vi "init.vi"(8 "error in (no error)":errorcluster, 9 "Image Type":T1=1 items=["Grayscale (U8)", "Grayscale (I16)", "Grayscale (SGL)", "Complex (CSG)", "RGB (U32)", "HSL (U32)", "RGB (U64)", "Grayscale (U16)"], 10 "Camera Name":refnum<k21> caption="IMAQdx Session", 11 "ax5 in":refnum<class "ax5.lvclass">) -> (0 "error out":errorcluster, 3 "ax5 out":refnum<class "ax5.lvclass">)   [LabVIEW 2017, in "ax5.lvclass"]
uses:
  ax5.lvclass
  \\psf\Home/Desktop/Elkhorn Test/Elkhorn Test/JSONRPC Server Framework Examples/builds/JSON RPC over TCP/RT CompactRIO Target/My Source Distribution/home/lvuser/natinst/bin/methods/camera.lvclass
  camera.lvclass
  <resource>/objmgr/imaqdx.rc
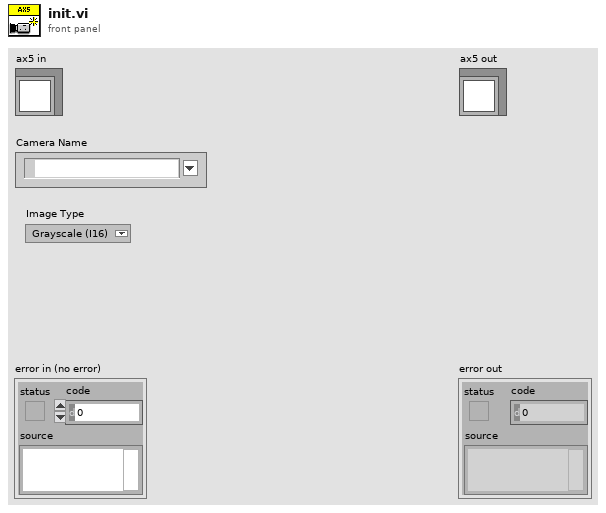
[diagram p1: front panel]
types:
  T1 = typedef "Image Type" = u32
  T2 = typedef "IMAQ Image.ctl" = refnum<image>
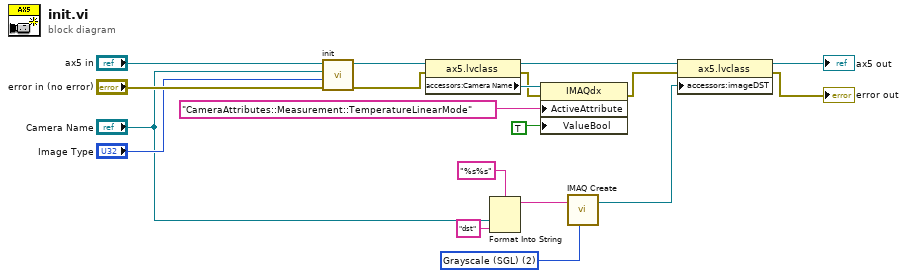
[diagram p0: block diagram]
diagram:
  w3 = T1 2 items=["Grayscale (U8)", "Grayscale (I16)", "Grayscale (SGL)", "Complex (CSG)", "RGB (U32)", "HSL (U32)", "RGB (U64)", "Grayscale (U16)"] ("Image Type")
  n1 = call-parent "init.vi"("error in (no error)"="error in (no error)", "Image Type"="Image Type", "Camera Name"="Camera Name", "camera in"="ax5 in") -> ("error out"=w15:errorcluster, "camera out"=w17:refnum<class "ax5.lvclass">)  [unwired: 6 in]
  n2 = property on="Property Node" class="ax5.lvclass"(reference=w17, error in=w15) -> (reference out=w10:refnum<class "ax5.lvclass">, error out=w9:errorcluster, "accessors:Camera Name"=w16:refnum<k21>)
  n3 = Format Into String(format string="%s%s", "Camera Name", "dst" ("input 2")) -> (resulting string=w5:string)  [unwired: 2 in, 1 out]
  n4 = property class="IMAQdx"(reference=w16, error in=w9, "ActiveAttribute"="CameraAttributes::Measurement::TemperatureLinearMode", "ValueBool"=TRUE) -> (error out=w11:errorcluster)  [unwired: 1 out]
  n5 = call "IMAQ Create"("Image Name"=w5, "Image Type"=w3) -> ("New Image"=w4:T2)  [unwired: 2 in, 2 out]
  n6 = property class="ax5.lvclass"(reference=w10, error in=w11, "accessors:imageDST"=w4) -> (reference out=→"ax5 out":refnum<class "ax5.lvclass">, error out=→"error out":errorcluster)
